vi "Create from Session.vi"(8 "Error In":errorcluster, 11 "Session In":refnum<class "Session.lvclass">) -> (0 "Error Out":errorcluster, 2 "File Info":refnum<class "File Info.lvclass">, 3 "Session Out":refnum<class "Session.lvclass">)   [LabVIEW 2021, in "Field_RnD_Services_LIBSSH2_Toolkit.lvlib" / "File Info.lvclass"]
doc: "Passes through the Session object but obtains the SSH context for the Session object to create a new File Info object."
uses:
  File Info.lvclass
  Session/Session.lvclass
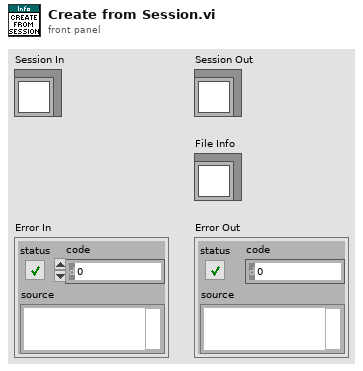
[diagram p1: front panel]
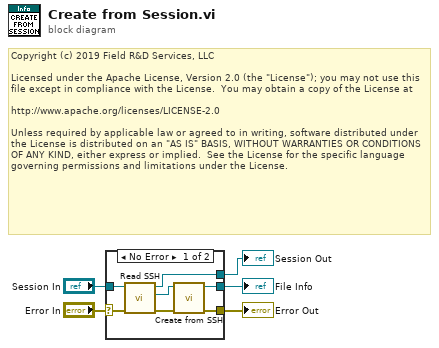
[diagram p0: block diagram]
diagram:
  # "Copyright (c) 2019 Field R&D Services, LLC\n\nLicensed under the Apache License, Version 2.0 (the \"License\"); you may not use this file except in compliance with the License.  You may obtain a copy of the License at\n\nhttp://www.apache.org/licenses/LICENSE-2.0\n\nUnless required by applicable law or agreed to in writing, software distributed under the License is distributed on an \"AS IS\" BASIS, WITHOUT WARRANTIES OR CONDITIONS OF ANY KIND, either express or implied.  See the License for the specific language governing permissions and limitations under the License."
  n1 = case shown="No Error" "Error In" {
    selector: "Error In" -> [w11 w14]
    tunnel: [w6 w14] -> w4
    tunnel: "Session In" -> [w12 w13]
    tunnel: [w9 w13] -> w2
    tunnel: [w8 _] -> w1
    frame No Error {
      n2 = call "Read SSH.vi"("Error In"=w11, "Session In"=w12) -> ("Erorr Out"=w7:errorcluster, "SSH"=w10:refnum<class "SSH.lvclass">, "Session Out"=w9:refnum<class "Session.lvclass">)  [unwired: 7 in]
      n3 = call "Create from SSH.vi"("Error In"=w7, "SSH"=w10) -> ("Error Out"=w6:errorcluster, "File Info"=w8:refnum<class "File Info.lvclass">)  [unwired: 8 in]
    }
    frame Error {
    }
  }
  "Error Out" <- w4
  "File Info" <- w1
  "Session Out" <- w2
